vi "json Insert Path - string path.vi"(8 "error in (no error)":errorcluster, 9 "anything":path, 10 "path":string, 11 "JSON Document in":refnum<class "JSON Document.lvclass">) -> (0 "error out":errorcluster, 1 "replaced?":bool, 3 "JSON Document out":refnum<class "JSON Document.lvclass">)   [LabVIEW 2015, in "JSON Document.lvclass"]
uses:
  JSON Document.lvclass
  JSON Document.lvclass/JSON Document.ctl
  rapidjson wrapper/rapidjson wrapper.lvlib
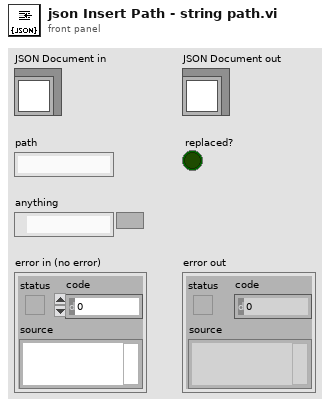
[diagram p1: front panel]
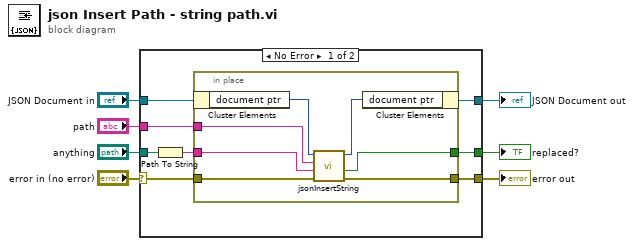
[diagram p0: block diagram]
diagram:
  n1 = case shown="No Error" "error in (no error)" {
    selector: "error in (no error)" -> [w11 w24]
    tunnel: [w12 w24] -> w6
    tunnel: [w14 w23] -> w4
    tunnel: "JSON Document in" -> [w15 w23]
    tunnel: "anything" -> [w10 _]
    tunnel: "path" -> [w13 _]
    tunnel: [w8 _] -> w1
    frame No Error {
      n2 = Path To String(path=w10) -> (string=w9:string)
      n3 = in-place {
        in-place-border: w13 -> [w17]
        in-place-border: w11 -> [w21]
        in-place-border: [w20] -> w12
        in-place-border: w9 -> [w19]
        in-place-border: [w16] -> w8
        n4 = in-place-cluster #1(w15) -> ("document ptr"=w18:i64)
        n5 = call "jsonInsertString.vi"("error in (no error)"=w21, "value"=w19, "path"=w17, "d in"=w18) -> ("error out"=w20:errorcluster, "replaced?"=w16:bool, "d out"=w22:i64)  [unwired: 5 in]
        n6 = in-place-cluster #1("document ptr"=w22) -> (w14:refnum<class "JSON Document.lvclass">)
      }
    }
    frame Error {
    }
  }
  "error out" <- w6
  "JSON Document out" <- w4
  "replaced?" <- w1
